vi "소켓 연습_시연본.vi"() -> ()   [LabVIEW 2023]
panel:
  out "e":i32
  out "theta":i32
  in  "stop 4":bool
  out "전체 Array":i32[](array[numeric])=[99, 99, 0, 0, 0, 0]
  out "data out":string="99,99,0,0,0,0"
  in  "stop 3":bool
  in  "stop 2":bool
  in  "stop":bool
  out "생산자 FPS":dbl=100.0 format="%#_2g"
  out "error out":errorcluster
  # "신호등 카메라 맨위,오른쪽 기준 줌50 좌7 아래12"
  # "배달 줌 25퍼 좌 끝 위아래는 중앙"
  # "파이썬에서 socket 통해 받아온 raw data"
  # "parsing 통해 Array 추출하는데 인덱스 0,1은 인식되는 신호등 클래스 번호. 여기서 0은 빨간불, 1은 좌회전, 2는 직진 ,99는 null 값이라 무시\n인덱스 2~4는 배달 표지판인데 아직 파이썬 코드 미완성(듀얼 스크린 불가)로 인해 0으로 뜸."
  # "전체 인덱스에서 신호등 인덱스만 따로 보이게 자름"
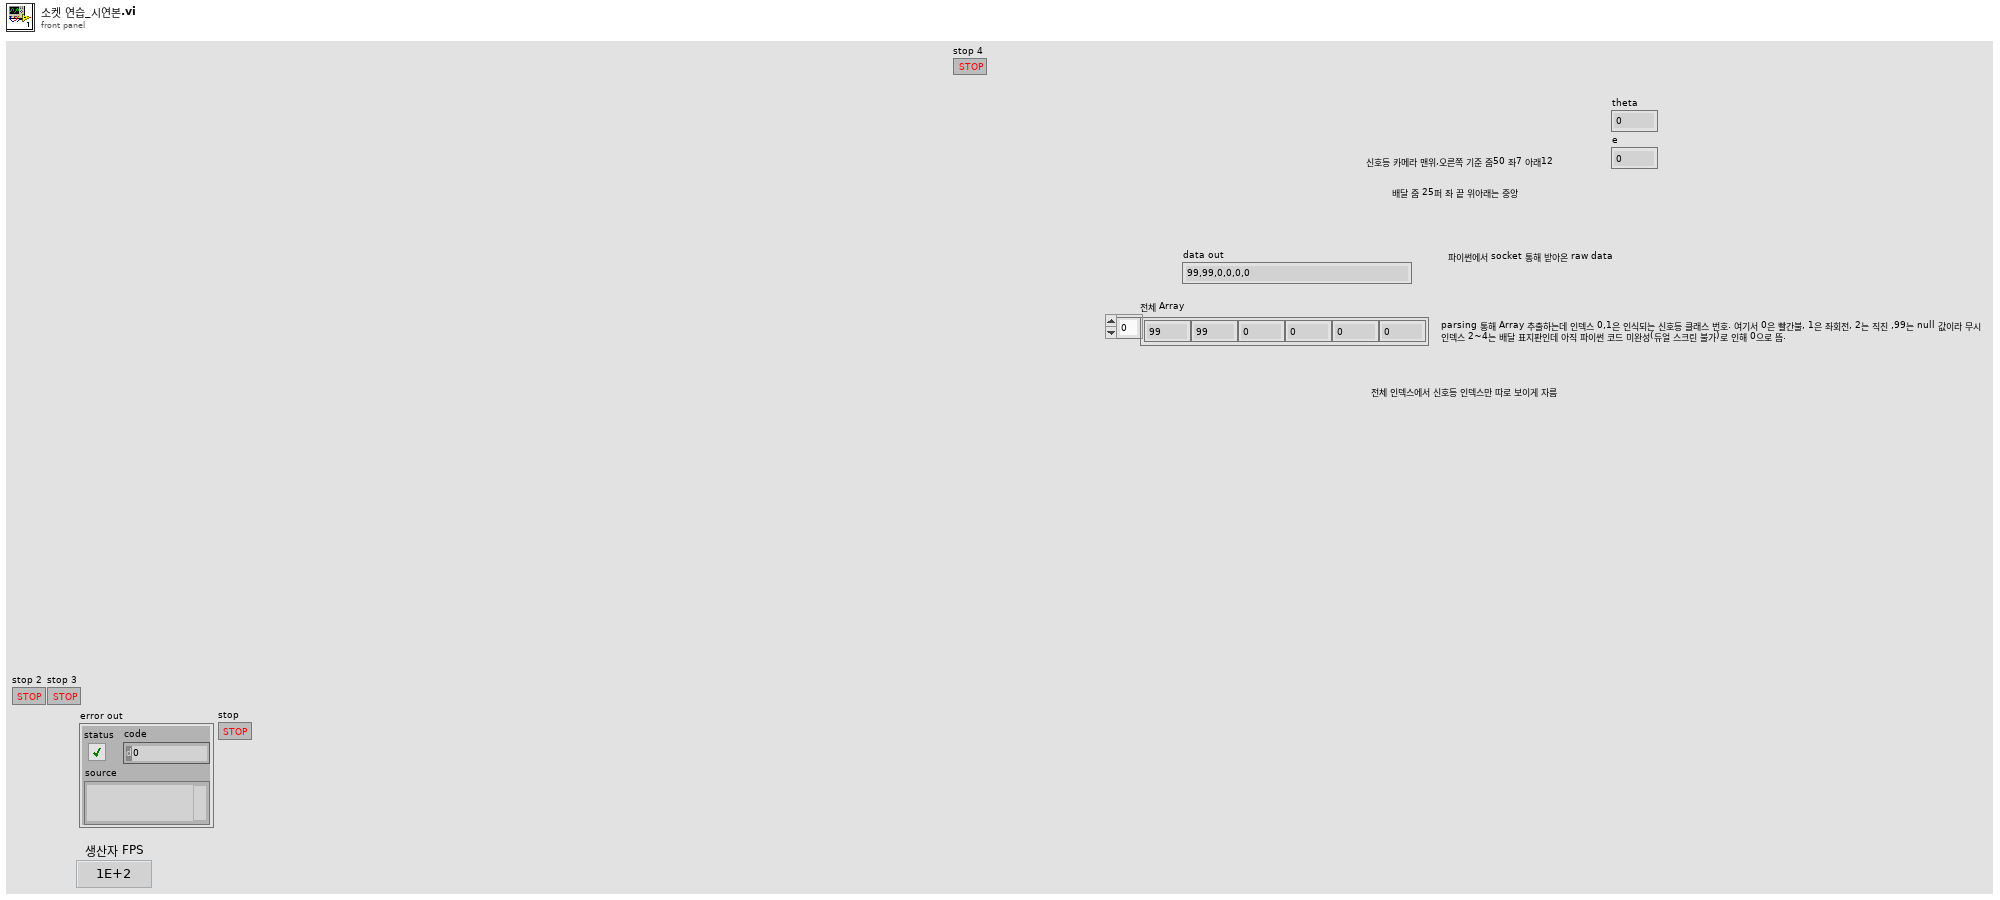
[diagram p1: front panel]
types:
  T1 = enum16{"Standard", "Buffered", "CRLF", "Immediate"}
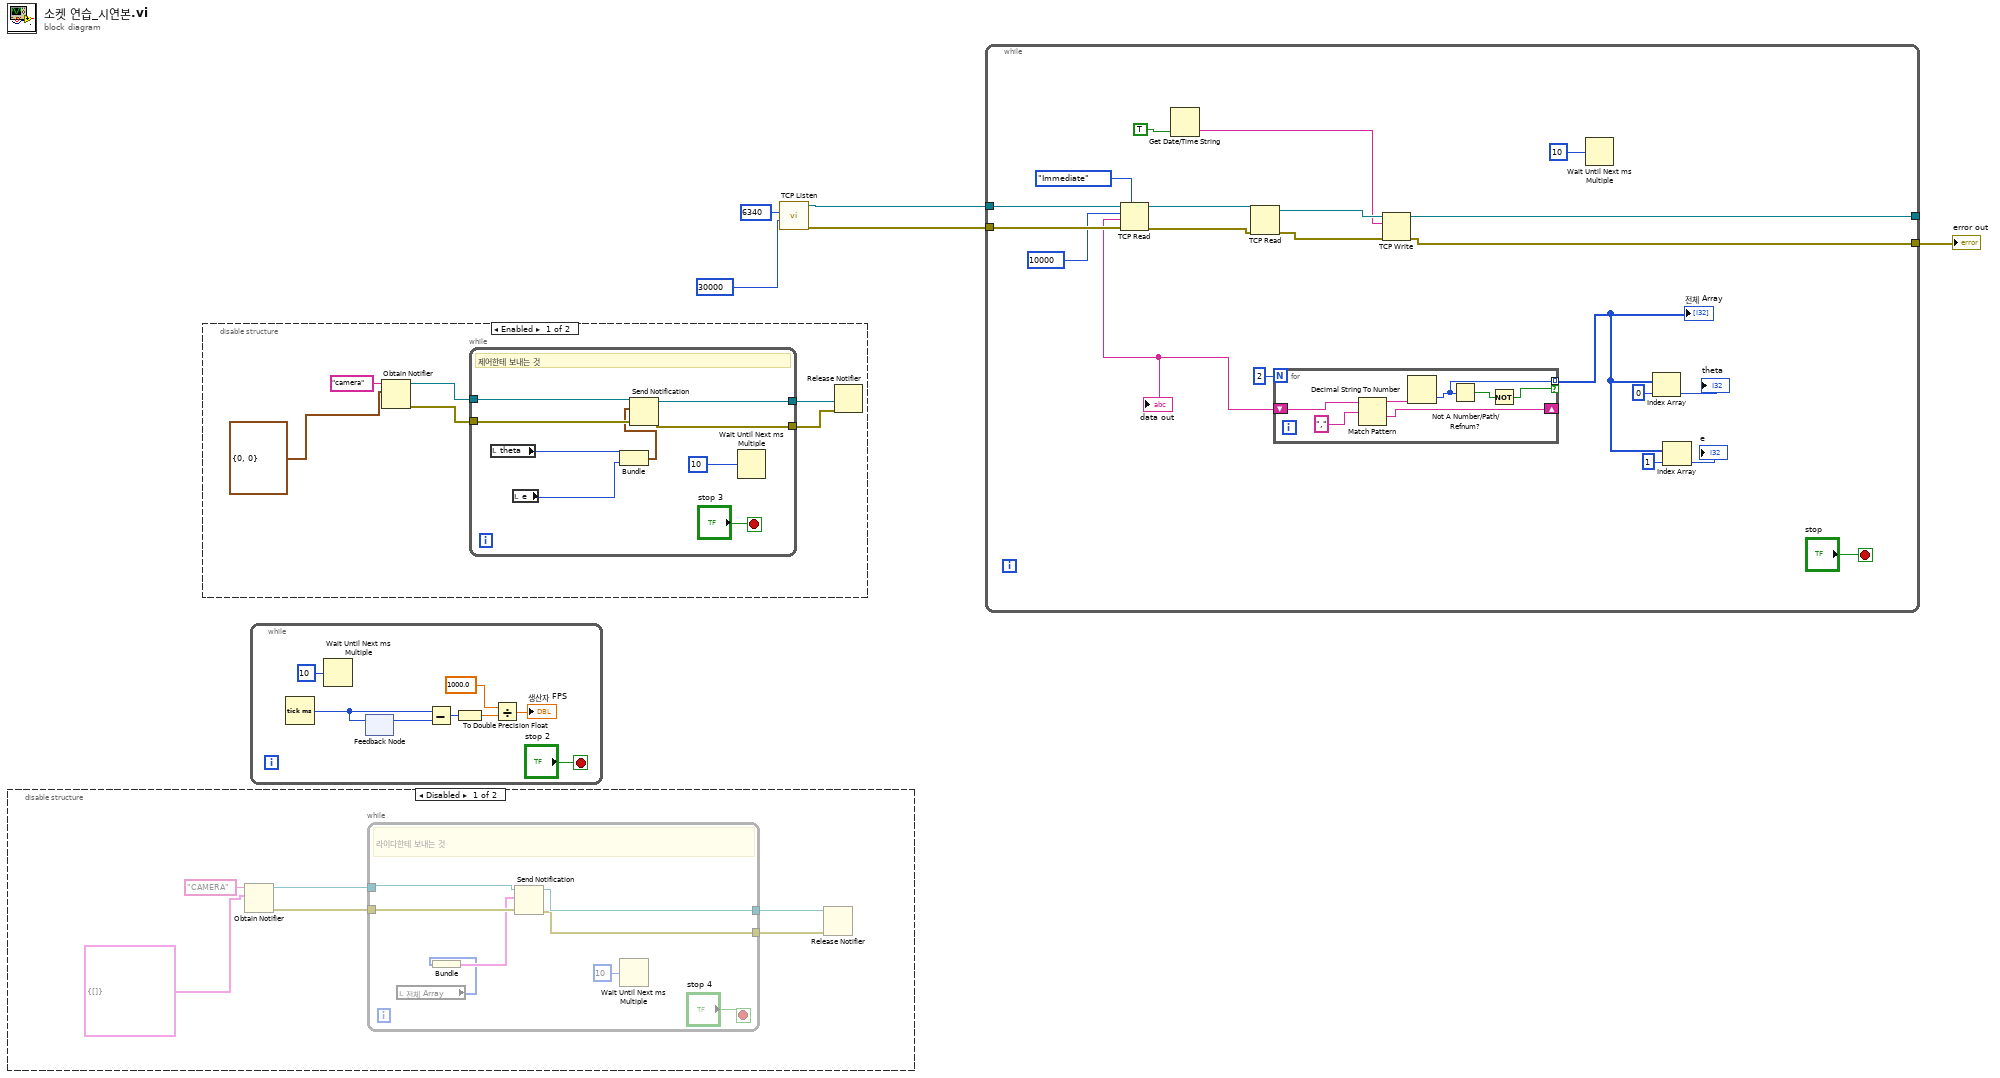
[diagram p0: block diagram]
diagram:
  n1 = disable-structure shown="Disabled" {
    frame Disabled {
      n2 = Obtain Notifier(name (unnamed)="CAMERA", notification data type=cluster{i32[]} {[]}) -> (notifier out=w11:refnum<notifier>, error out=w8:errorcluster)  [unwired: 2 in, 1 out]
      n3 = while {
        tunnel: w11 -> [w19]
        tunnel: w8 -> [w18]
        tunnel: [w15] -> w7
        tunnel: [w14] -> w6
        stop <- "stop 4" stop-if-true
        # "라이다한테 보내는 것"
        n4 = local read "전체 Array"() -> (w16:i32[])
        n5 = Bundle("전체 Array"=w16) -> (w17:cluster{"전체 Array":i32[]})  [unwired: 1 in]
        n6 = Send Notification(notification=w17, notifier=w19, error in (no error)=w18) -> (notifier out=w15:refnum<notifier>, error out=w14:errorcluster)
        n7 = Wait Until Next ms Multiple(millisecond multiple=u32 10) -> ()  [unwired: 1 out]
      }
      n8 = Release Notifier(notifier=w7, error in (no error)=w6) -> ()  [unwired: 1 in, 3 out]
    }
    frame Enabled {
    }
  }
  n9 = disable-structure shown="Enabled" {
    frame Enabled {
      n10 = Obtain Notifier(name (unnamed)="camera", notification data type=cluster{i32, i32} {0, 0}) -> (notifier out=w25:refnum<notifier>, error out=w23:errorcluster)  [unwired: 2 in, 1 out]
      n11 = while {
        tunnel: w25 -> [w34]
        tunnel: w23 -> [w33]
        tunnel: [w32] -> w22
        tunnel: [w31] -> w21
        stop <- "stop 3" stop-if-true
        # "제어한테 보내는 것"
        n12 = local read "theta"() -> (w28:i32)
        n13 = local read "e"() -> (w27:i32)
        n14 = Bundle("theta"=w28, "e"=w27) -> (w26:cluster{"theta":i32, "e":i32})  [unwired: 1 in]
        n15 = Send Notification(notification=w26, notifier=w34, error in (no error)=w33) -> (notifier out=w32:refnum<notifier>, error out=w31:errorcluster)
        n16 = Wait Until Next ms Multiple(millisecond multiple=u32 10 ("milliseconds to wait")) -> ()  [unwired: 1 out]
      }
      n17 = Release Notifier(notifier=w22, error in (no error)=w21) -> ()  [unwired: 1 in, 3 out]
    }
    frame Disabled {
    }
  }
  n18 = while {
    stop <- "stop 2" stop-if-true
    n19 = Tick Count (ms)() -> (millisecond timer value=w40:u32)
    n20 = Wait Until Next ms Multiple(millisecond multiple=u32 10 ("ms 배수")) -> ()  [unwired: 1 out]
    n21 = feedback #1() -> (w41:u32)  [unwired: 1 in]
    n22 = feedback-in #1(w40) -> ()
    n23 = Subtract(x=w40, y=w41) -> (x-y=w42:u32)
    n24 = To Double Precision Float(number=w42) -> (double precision float=w39:dbl)
    n25 = Divide(x=1000.0, y=w39) -> (x/y=→"생산자 FPS":dbl)
  }
  n26 = call <vilib>:"TCP Listen.vi"("timeout ms (wait forever: -1)"=30000, "port"=u16 6340) -> ("error out"=w2:errorcluster, "connection ID"=w5:refnum<k5>)  [unwired: 5 in, 3 out]
  n27 = while {
    tunnel: w5 -> [w63]
    tunnel: w2 -> [w62]
    tunnel: [w53] -> w1
    tunnel: [w52] -> _
    stop <- "stop" stop-if-true
    n28 = TCP Read(connection ID=w63, bytes to read=10000, error in (no error)=w62, 7:T1."Immediate" ("mode (standard)")) -> (connection ID out=w59:refnum<k5>, data out=w48:string, error out=w58:errorcluster)  [unwired: 1 in]
    "data out" <- w48
    n29 = Get Date/Time String(want seconds? (F)=TRUE) -> (time string=w54:string)  [unwired: 2 in, 1 out]
    n30 = TCP Read(connection ID=w59, error in (no error)=w58) -> (connection ID out=w57:refnum<k5>, error out=w56:errorcluster)  [unwired: 3 in, 1 out]
    n31 = for {
      N: 2 -> [_]
      tunnel: [w66] -> w43 mode=indexing if=w64
      shift-right: [w67] -> _
      shift-left: w48 -> [w70]
      n32 = Match Pattern(string=w70, regular expression=",") -> (before substring=w68:string, after substring=w67:string)  [unwired: 1 in, 2 out]
      n33 = Decimal String To Number(string=w68) -> (number=w66:i32)  [unwired: 2 in, 1 out]
      n34 = Not A Number/Path/Refnum?(number/path/refnum=w66) -> (NaN/Path/Refnum?=w65:bool)
      n35 = Not(x=w65) -> (.not. x?=w64:bool)
    }
    "전체 Array" <- w43
    n36 = TCP Write(connection ID=w57, data in=w54, error in (no error)=w56) -> (connection ID out=w52:refnum<k5>, error out=w53:errorcluster)  [unwired: 1 in, 1 out]
    n37 = Wait Until Next ms Multiple(millisecond multiple=u32 10) -> ()  [unwired: 1 out]
    n38 = Index Array(array=w43, index=0) -> (element=→"theta":i32)
    n39 = Index Array(array=w43, index=1) -> (element=→"e":i32)
  }
  "error out" <- w1
